vi "Populate Project Ring.vi"(8 "Error In":errorcluster, 11 "State In":T1) -> (0 "Error Out":errorcluster, 3 "State Out":T1)   [LabVIEW 2018, in "Bookmark Manager.lvlib"]
uses:
  Bookmark Manager.lvlib
  Controls/State.ctl
  <vilib>/addons/analyzer/_analyzerctrls.llb/VIAnCtl Analysis App Info.ctl
  Controls/Bookmark.ctl
  Controls/VI Identifier.ctl
  Controls/Bookmarks Groups.ctl
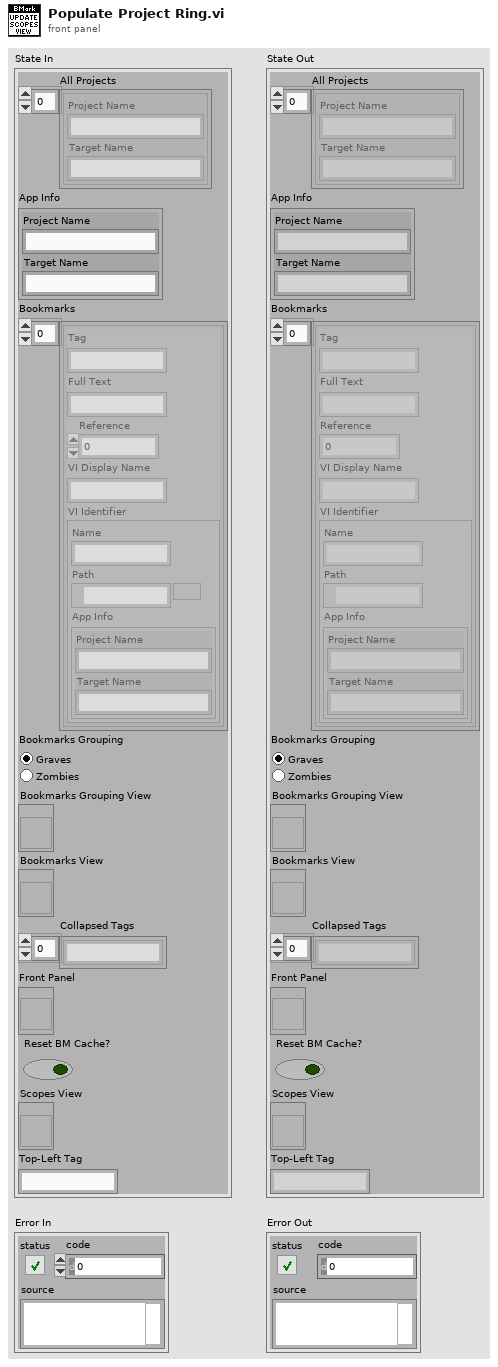
[diagram p1: front panel]
types:
  T1 = typedef "Bookmark Manager.lvlib/State.ctl" = cluster{"All Projects":T2[], "App Info":T2, "Bookmarks":T3[], "Bookmarks Grouping":T5, "Bookmarks Grouping View":refnum<vi>, "Bookmarks View":refnum<vi>, "Collapsed Tags":string[], "Front Panel":refnum<vi>, "Reset BM Cache?":bool, "Scopes View":refnum<vi>, "Top-Left Tag":string}
  T2 = typedef "VIAnCtl Analysis App Info.ctl" = cluster{"Project Name":string, "Target Name":string}
  T3 = typedef "Bookmark Manager.lvlib/Bookmark.ctl" = cluster{"Tag":string, "Full Text":string, "Reference":i32, "VI Display Name":string, "VI Identifier":T4}
  T4 = typedef "Bookmark Manager.lvlib/VI Identifier.ctl" = cluster{"Name":string, "Path":path, "App Info":T2}
  T5 = typedef "Bookmark Manager.lvlib/Bookmarks Groups.ctl" = enum32{"Graves", "Zombies"}
  T6 = enum8{"Enabled", "Disabled", "Disabled and Grayed Out"}
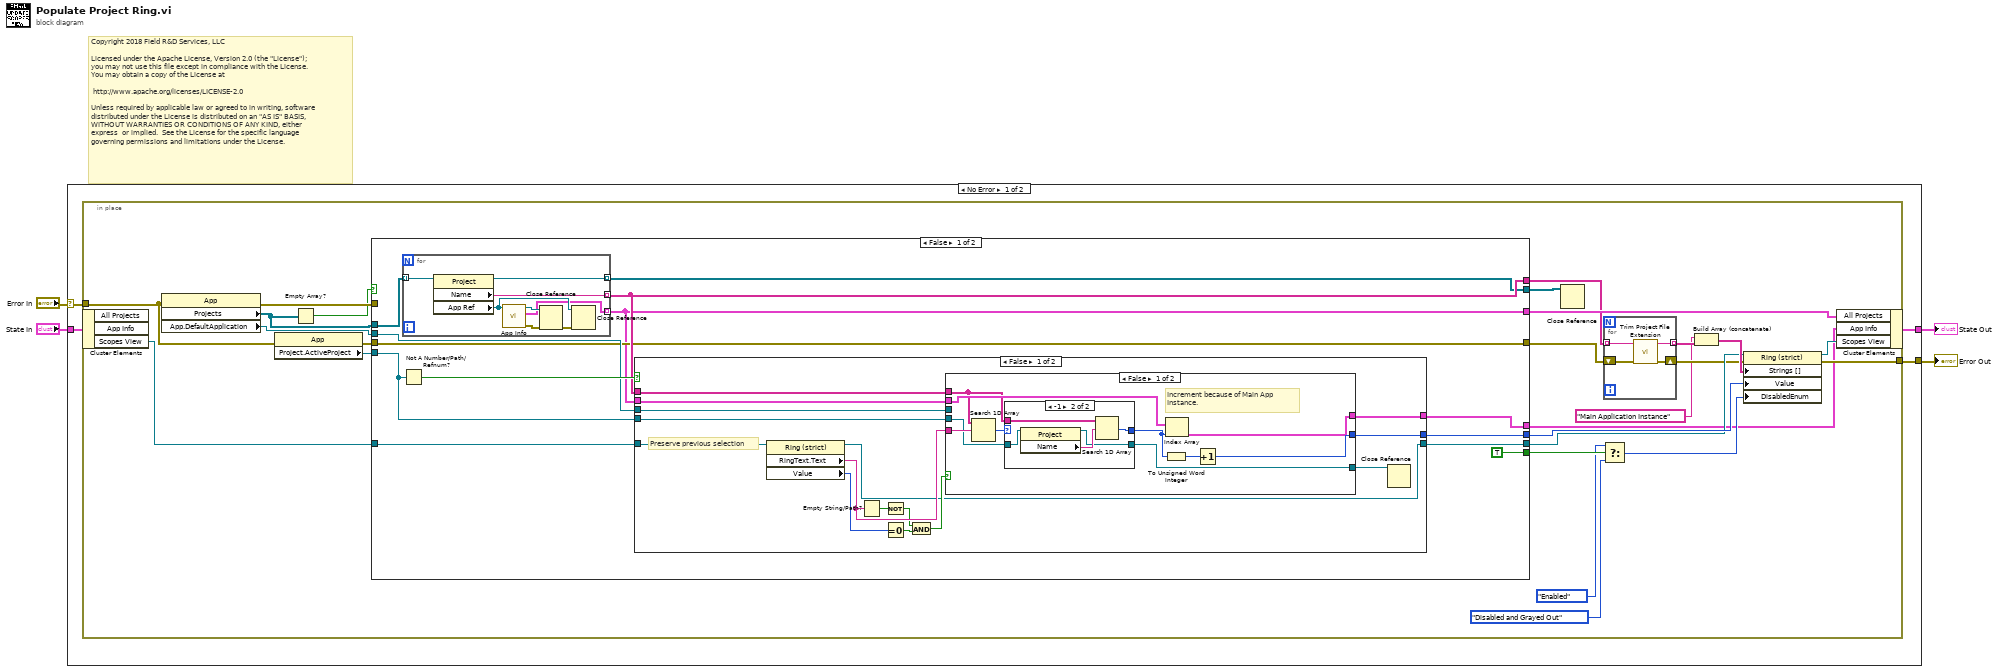
[diagram p0: block diagram]
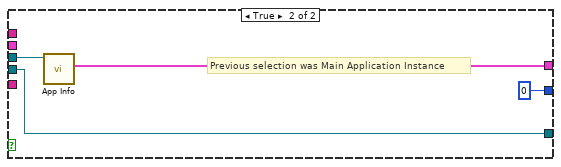
[diagram p3: hidden frame]
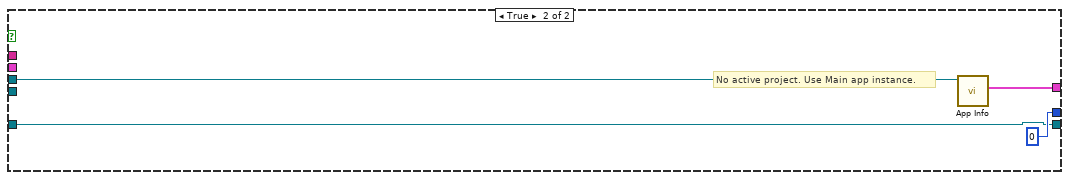
[diagram p4: hidden frame]
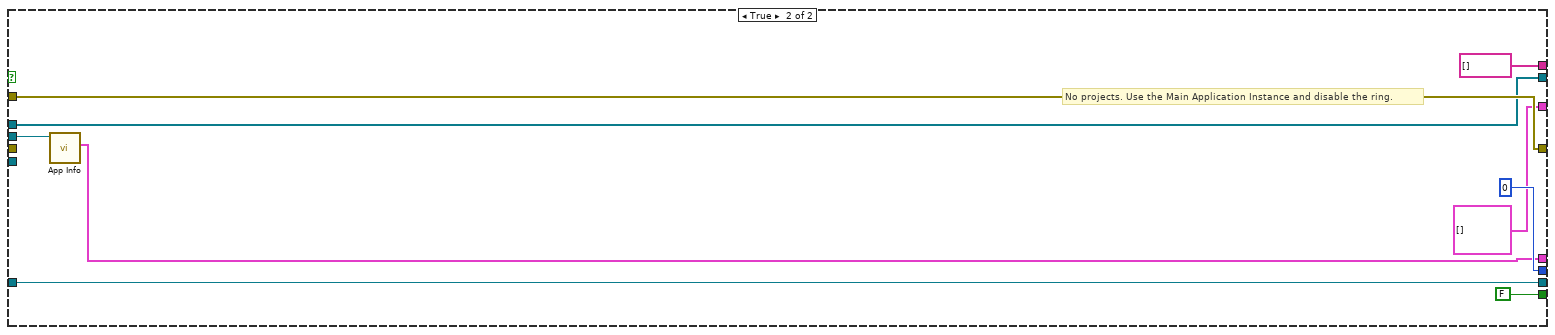
[diagram p5: hidden frame]
diagram:
  # "Copyright 2018 Field R&D Services, LLC\n\nLicensed under the Apache License, Version 2.0 (the \"License\");\nyou may not use this file except in compliance with the License.\nYou may obtain a copy of the License at\n\n\thttp://www.apache.org/licenses/LICENSE-2.0\n\nUnless required by applicable law or agreed to in writing, software\ndistributed under the License is distributed on an \"AS IS\" BASIS,\nWITHOUT WARRANTIES OR CONDITIONS OF ANY KIND, either \nexpress  or implied.  See the License for the specific language \ngoverning permissions and limitations under the License."
  n1 = case shown="No Error" "Error In" {
    selector: "Error In" -> [w5 w109]
    tunnel: [w8 w109] -> w4
    tunnel: "State In" -> [w7 w108]
    tunnel: [w6 w108] -> w2
    frame No Error {
      n2 = in-place {
        in-place-border: [w33] -> w8
        in-place-border: w5 -> [w32]
        n3 = in-place-cluster #1(w7) -> ("Scopes View"=w17:refnum<vi>)  [unwired: 2 out]
        n4 = property class="App"(error in=w32) -> (error out=w27:errorcluster, "Projects"=w26:refnum<vi>[], "App.DefaultApplication"=w28:refnum<vi>)  [unwired: 1 in, 1 out]
        n5 = property class="App"(error in=w32) -> (error out=w31:errorcluster, "Project.ActiveProject"=w29:refnum<vi>)  [unwired: 1 in, 1 out]
        n6 = Empty Array?(array=w26) -> (empty?=w25:bool)
        n7 = case shown="False" w25 {
          tunnel: [w43 w107] -> w12
          tunnel: w31 -> [w43 _]
          tunnel: [TRUE FALSE] -> w22
          tunnel: [w47 string[] []] -> w13
          tunnel: [w41 T2[] [] ("all projects")] -> w15
          tunnel: [w46 u16 0] -> w30
          tunnel: w26 -> [w44 w101]
          tunnel: w29 -> [w49 _]
          tunnel: w28 -> [w45 w102]
          tunnel: [w40 w100] -> w14
          tunnel: w27 -> [_ w107]
          tunnel: [w42 w101] -> w19
          tunnel: [w39 w99] -> w18
          tunnel: w17 -> [w38 w99]
          frame False {
            n8 = Not A Number/Path/Refnum?(number/path/refnum=w49) -> (NaN/Path/Refnum?=w48:bool)
            n9 = for {
              tunnel: w44 -> [w97] mode=indexing
              tunnel: [w91] -> w47 mode=indexing
              tunnel: [w98] -> w42 mode=indexing
              tunnel: [w92] -> w41 mode=indexing
              n10 = property class="Project"(reference=w97) -> (reference out=w98:refnum<vi>, "Name"=w91:string, "App Ref"=w94:refnum<vi>)  [unwired: 1 in, 1 out]
              n11 = call "App Info.vi"("App Refnum"=w94) -> ("Error Out"=w96:errorcluster, "App Info"=w92:T2, "App Refnum for Opening VI"=w93:refnum<vi>)  [unwired: 8 in]
              n12 = Close Reference(reference=w93, error in (no error)=w96) -> (error out=w95:errorcluster)
              n13 = Close Reference(reference=w94, error in (no error)=w95) -> ()  [unwired: 1 out]
            }
            n14 = case shown="False" w48 {
              tunnel: w47 -> [w62 _]
              tunnel: w49 -> [w63 _]
              tunnel: [w64 u16 0] -> w46
              tunnel: w41 -> [w65 _]
              tunnel: w45 -> [w60 w89]
              tunnel: [w61 w88] -> w40
              tunnel: [w52 w87] -> w39
              tunnel: w38 -> [w51 w87]
              frame False {
                # "Preserve previous selection"
                n15 = property class="Ring (strict)"(reference=w51) -> (reference out=w52:refnum<vi>, "RingText.Text"=w56:string, "Value"=w58:u16)  [unwired: 1 in, 1 out]
                n16 = Empty String/Path?(string/path=w56) -> (empty?=w57:bool)
                n17 = Not(x=w57) -> (.not. x?=w53:bool)
                n18 = Equal To 0?(x=w58) -> (x = 0?=w55:bool)
                n19 = And(x=w53, y=w55) -> (x .and. y?=w54:bool)
                n20 = case shown="False" w54 {
                  tunnel: w65 -> [w75 _]
                  tunnel: w56 -> [w74 _]
                  tunnel: [w73 u16 0] -> w64
                  tunnel: w63 -> [w70 w84]
                  tunnel: w62 -> [w69 _]
                  tunnel: [w68 w83] -> w61
                  tunnel: w60 -> [_ w86]
                  tunnel: [w67 w84] -> w59
                  frame False {
                    # "Increment because of Main App Instance."
                    n21 = Search 1D Array(1D array=w69, element=w74) -> (index of element=w66:i32)  [unwired: 1 in]
                    n22 = case shown="-1" w66 {
                      selector: w66 -> [w76 _]
                      tunnel: [w76 w80] -> w71
                      tunnel: w70 -> [w77 w82]
                      tunnel: w69 -> [_ w79]
                      tunnel: [w77 w78] -> w67
                      frame Default {
                      }
                      frame -1 {
                        n23 = property class="Project"(reference=w82) -> (reference out=w78:refnum<vi>, "Name"=w81:string)  [unwired: 1 in, 1 out]
                        n24 = Search 1D Array(1D array=w79, element=w81) -> (index of element=w80:i32)  [unwired: 1 in]
                      }
                    }
                    n25 = To Unsigned Word Integer(number=w71) -> (unsigned 16bit integer=w72:u16)
                    n26 = Index Array(array=w75, index=w71) -> (element=w68:T2)
                    n27 = Increment(x=w72) -> (x+1=w73:u16)
                  }
                  frame True {
                    # "Previous selection was Main Application Instance"
                    n28 = call "App Info.vi"("App Refnum"=w86) -> ("App Info"=w83:T2)  [unwired: 8 in, 2 out]
                  }
                }
                n29 = Close Reference(reference=w59) -> ()  [unwired: 1 in, 1 out]
              }
              frame True {
                # "No active project. Use Main app instance."
                n30 = call "App Info.vi"("App Refnum"=w89) -> ("App Info"=w88:T2)  [unwired: 8 in, 2 out]
              }
            }
          }
          frame True {
            # "No projects. Use the Main Application Instance and disable the ring."
            n31 = call "App Info.vi"("App Refnum"=w102) -> ("App Info"=w100:T2)  [unwired: 8 in, 2 out]
          }
        }
        n32 = Close Reference(reference=w19) -> ()  [unwired: 1 in, 1 out]
        n33 = Select(t=T6."Enabled" ("Disabled"), s=w22, f=T6."Disabled and Grayed Out" ("Disabled")) -> (s? t:f=w20:T6)
        n34 = for {
          tunnel: w13 -> [w37] mode=indexing
          shift-right: [w35] -> w11
          shift-left: w12 -> [w36]
          tunnel: [w34] -> w10 mode=indexing
          n35 = call "Trim Project File Extension.vi"("Error In"=w36, "Project File Name"=w37) -> ("Error Out"=w35:errorcluster, "Project Name"=w34:string)  [unwired: 8 in]
        }
        n36 = Build Array (concatenate)("Main Application Instance", w10) -> (w24:string[])
        n37 = property on="Property Node" class="Ring (strict)"(reference=w18, error in=w11, "Strings []"=w24, "Value"=w30, "DisabledEnum"=w20) -> (reference out=w16:refnum<vi>, error out=w33:errorcluster)
        n38 = in-place-cluster #1("All Projects"=w15, "App Info"=w14, "Scopes View"=w16) -> (w6:T1)
      }
    }
    frame Error {
    }
  }
  "Error Out" <- w4
  "State Out" <- w2
